vi "Constant - Blank Module Data.vi"() -> (0 "Blank Module Data":T1)   [LabVIEW 2016, in "Error Manager.lvlib"]
doc: "Blank VI with error handling."
uses:
  Error Manager.lvlib
  Read-Unread Status (enum).ctl
  Display Order (enum).ctl
  Error in current one-second interval (cluster).ctl
  Module Data (cluster).ctl
  Handled Error (cluster).ctl
  GUI Object References (cluster).ctl
panel:
  # "Input\nInputs to the VI"
  # "Development\nControls or indicators that are useful for development or testing, but which are not outputs of the VI."
  # "Output\nOutputs of the VI"
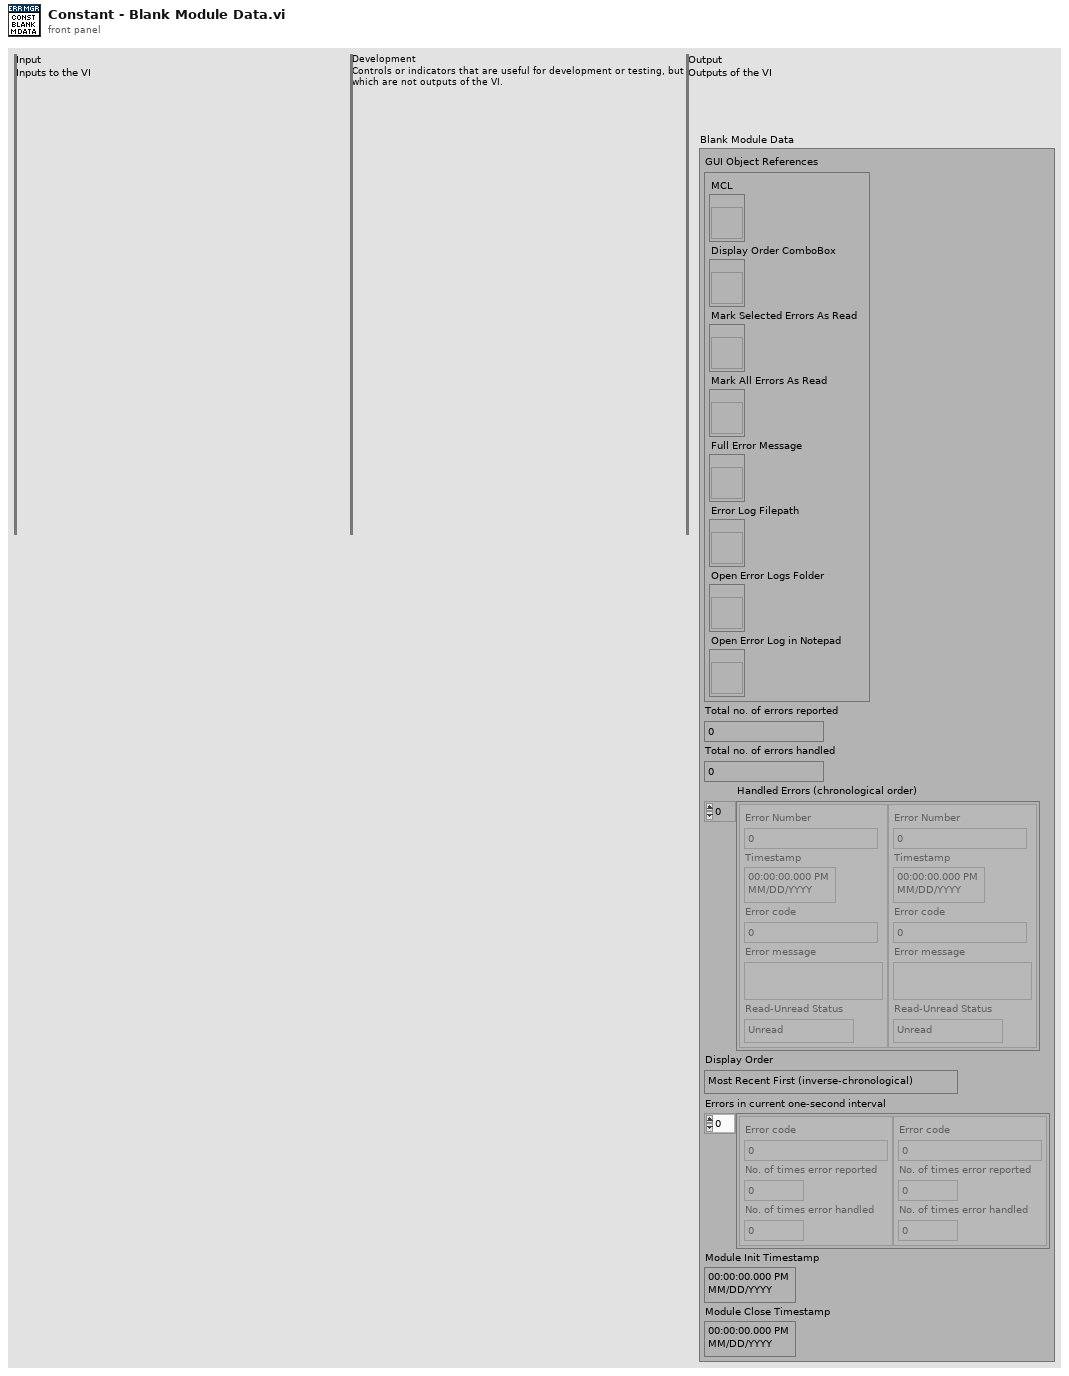
[diagram p1: front panel]
types:
  T1 = typedef "Error Manager.lvlib/Module Data (cluster).ctl" = cluster{"GUI Object References":T2, "Total no. of errors reported":i32, "Total no. of errors handled":i32, "Handled Errors (chronological order)":T3[], "Display Order":T5, "Errors in current one-second interval":T6[], "Module Init Timestamp":timestamp, "Module Close Timestamp":timestamp}
  T2 = typedef "Error Manager.lvlib/GUI Object References (cluster).ctl" = cluster{"MCL":refnum<vi>, "Display Order ComboBox":refnum<vi>, "Mark Selected Errors As Read":refnum<vi>, "Mark All Errors As Read":refnum<vi>, "Full Error Message":refnum<vi>, "Error Log Filepath":refnum<vi>, "Open Error Logs Folder":refnum<vi>, "Open Error Log in Notepad":refnum<vi>}
  T3 = typedef "Error Manager.lvlib/Handled Error (cluster).ctl" = cluster{"Error Number":i32, "Timestamp":timestamp, "Error code":i32, "Error message":string, "Read-Unread Status":T4}
  T4 = typedef "Error Manager.lvlib/Read-Unread Status (enum).ctl" = enum16{"Unread", "Read"}
  T5 = typedef "Error Manager.lvlib/Display Order (enum).ctl" = enum16{"Most Recent First (inverse-chronological)", "Oldest First (chronological)"}
  T6 = typedef "Error Manager.lvlib/Error in current one-second interval (cluster).ctl" = cluster{"Error code":i32, "No. of times error reported":u32, "No. of times error handled":u32}
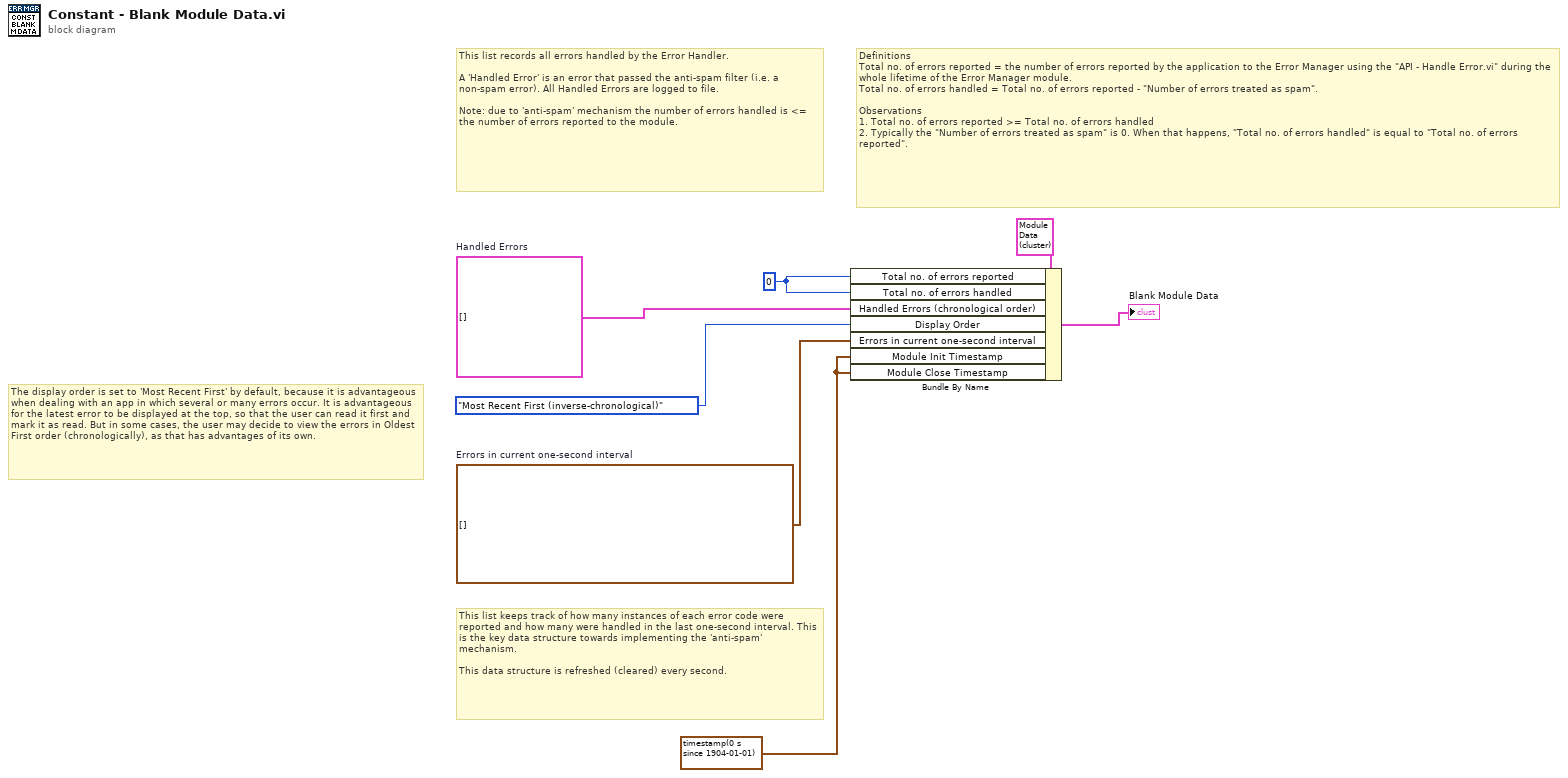
[diagram p0: block diagram]
diagram:
  w1 = timestamp(0 s since 1904-01-01) ("Module Init Timestamp")
  w2 = 0 ("Total no. of errors handled so far")
  w5 = T6[] []  # Errors in current one-second interval
  w7 = T3[] []  # Handled Errors
  # "Definitions\nTotal no. of errors reported = the number of errors reported by the application to the Error Manager using the \"API - Handle Error.vi\" during the whole lifetime of the Error Manager module.\nTotal no. of errors handled = Total no. of errors reported - \"Number of errors treated as spam\".\n\nObservations\n1. Total no. of errors reported >= Total no. of errors handled\n2. Typically the \"Number of errors treated as spam\" is 0. When that happens, \"Total no. of errors handled\" is equal to \"Total no. of errors reported\"."
  # "This list keeps track of how many instances of each error code were reported and how many were handled in the last one-second interval. This is the key data structure towards implementing the 'anti-spam' mechanism.\n\nThis data structure is refreshed (cleared) every second."
  # "This list records all errors handled by the Error Handler. \n\nA 'Handled Error' is an error that passed the anti-spam filter (i.e. a non-spam error). All Handled Errors are logged to file.\n\nNote: due to 'anti-spam' mechanism the number of errors handled is <= the number of errors reported to the module."
  # "The display order is set to 'Most Recent First' by default, because it is advantageous when dealing with an app in which several or many errors occur. It is advantageous for the latest error to be displayed at the top, so that the user can read it first and mark it as read. But in some cases, the user may decide to view the errors in Oldest First order (chronologically), as that has advantages of its own."
  n1 = Bundle By Name(cluster=T1 {"GUI Object References"={"MCL"=refnum, "Display Order ComboBox"=refnum, "Mark Selected Errors As Read"=refnum, "Mark All Errors As Read"=refnum, "Full Error Message"=refnum, "Error Log Filepath"=refnum, "Open Error Logs Folder"=refnum, "Open Error Log in Notepad"=refnum}, "Total no. of errors reported"=0, "Total no. of errors handled"=0, "Handled Errors (chronological order)"=[], "Display Order"=enum."Most Recent First (inverse-chronological)", "Errors in current one-second interval"=[], "Module Init Timestamp"=timestamp(0 s since 1904-01-01), "Module Close Timestamp"=timestamp(0 s since 1904-01-01)} ("Module Data"), "Total no. of errors reported"=w2, "Total no. of errors handled"=w2, "Handled Errors (chronological order)"=w7, "Display Order"=Display_Order_(enum)."Most Recent First (inverse-chronological)", "Errors in current one-second interval"=w5, "Module Init Timestamp"=w1, "Module Close Timestamp"=w1) -> (→"Blank Module Data":T1)
